vi "Ex8_Lissage_Signal.vi"() -> ()   [LabVIEW 2018]
panel:
  in  "stop":bool
  out "Graphe déroulant":cluster{dbl, dbl, dbl}(graph)
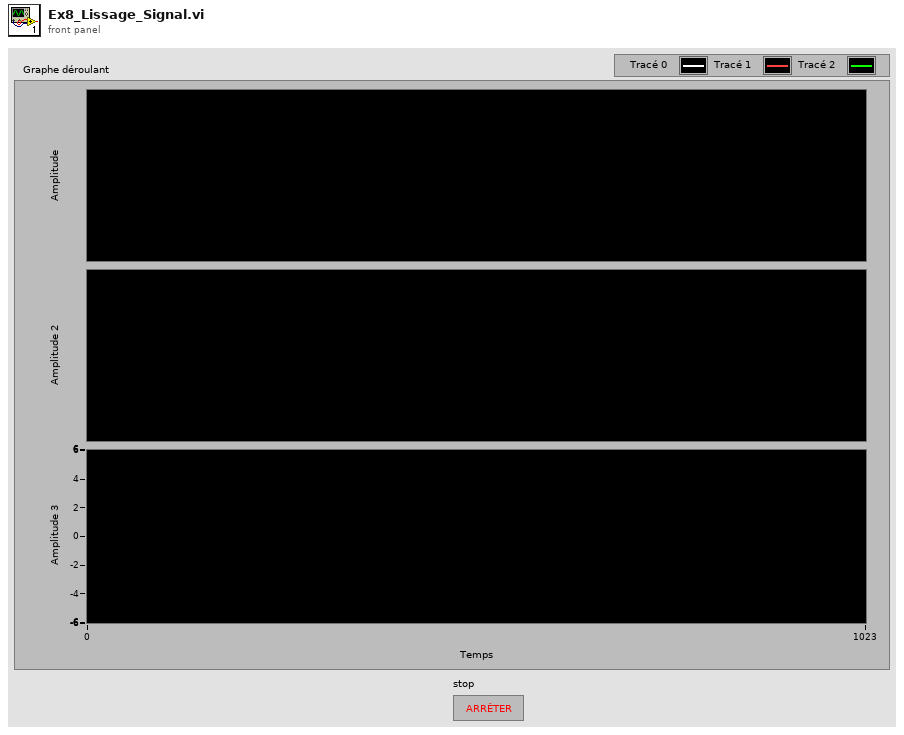
[diagram p1: front panel]
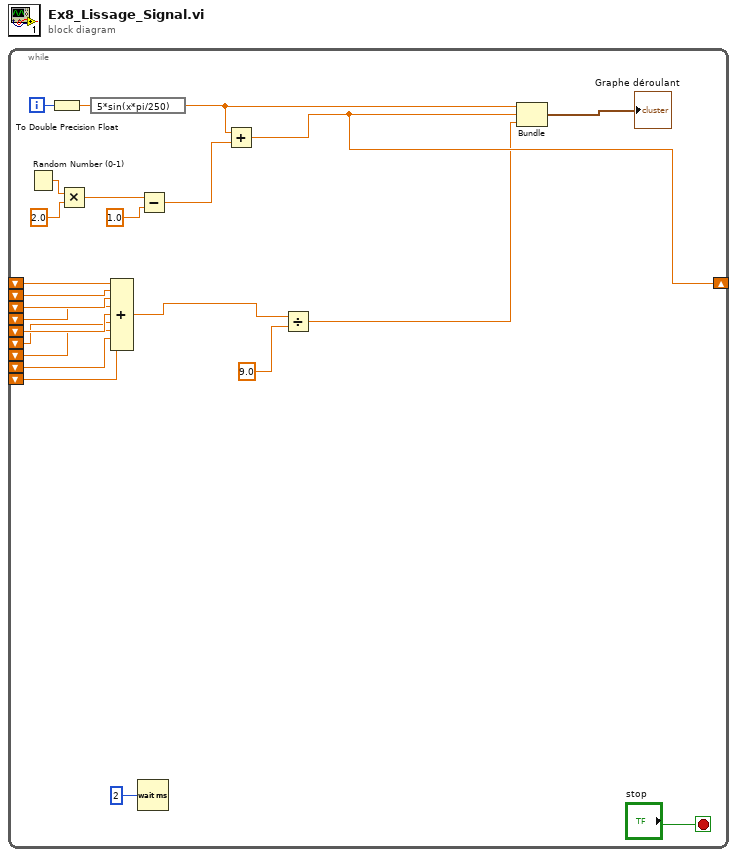
[diagram p0: block diagram]
diagram:
  n1 = while {
    shift-right: [w13] -> _
    shift-left: _ -> [w12]
    shift-left: _ -> [w11]
    shift-left: _ -> [w10]
    shift-left: _ -> [w9]
    shift-left: _ -> [w8]
    shift-left: _ -> [w7]
    shift-left: _ -> [w6]
    shift-left: _ -> [w5]
    shift-left: _ -> [w4]
    i -> [w21]
    stop <- "stop" stop-if-true
    n2 = Random Number (0-1)() -> (number: 0 to 1=w19:dbl)
    n3 = To Double Precision Float(number=w21) -> (double precision float=w23:dbl)
    n4 = Multiply(x=w19, y=2.0) -> (x*y=w17:dbl)
    n5 = expression code="5*sin(x*pi/250)"(w23) -> (w14:dbl)
    n6 = Compound Arithmetic op=ADD(w12, w11, w10, w9, w8, w7, w6, w5, w4) -> (w3:dbl)
    n7 = Wait (ms)(milliseconds to wait=u32 2 ("attente (ms)")) -> ()  [unwired: 1 out]
    n8 = Subtract(x=w17, y=1.0) -> (x-y=w15:dbl)
    n9 = Add(x=w14, y=w15) -> (x+y=w13:dbl)
    n10 = Divide(x=w3, y=9.0) -> (x/y=w1:dbl)
    n11 = Bundle(w14, w13, w1) -> (→"Graphe déroulant":cluster{dbl, dbl, dbl})  [unwired: 1 in]
  }
